vi "WSVCAP SHL Host TL RFFE Write Cycle.vi"(0 "RFFE Data Out":u8[][](array[numeric]) format="%.0x", 5 "Socket Mask":u64=1 format="%08x", 7 "Cycle CMD Lengths (bits)":u8[](array[numeric]), 9 "Cycle CMD Delay (ticks)":u32[](array[numeric]), 11 "error in":errorcluster, 13 "Log (T)":bool=TRUE, 14 "FPGA":T1) -> (15 "error out":errorcluster)   [LabVIEW 2012]
uses:
  Type Defs/WSVCAP SHL I2C FPGA Enum.ctl
  Type Defs/WSVCAP SHL Function Enum.ctl
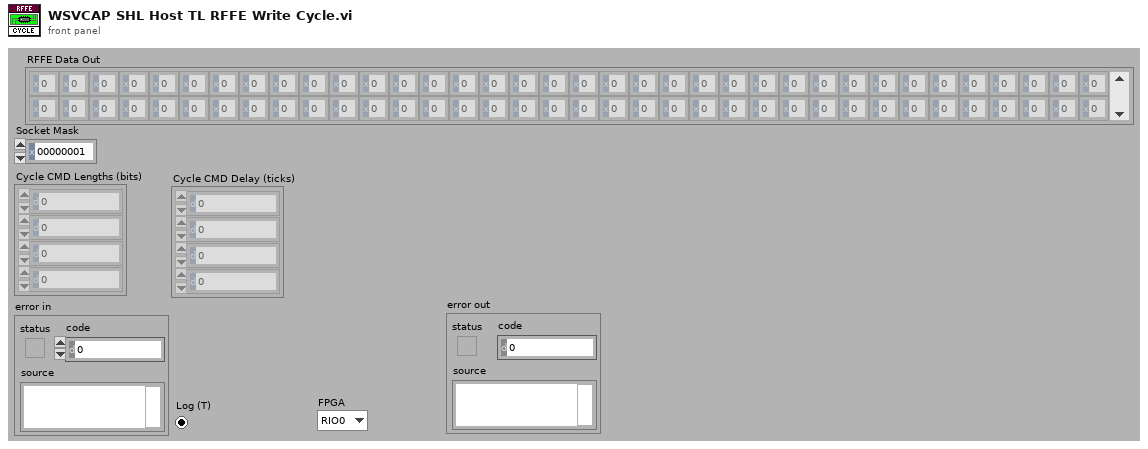
[diagram p1: front panel]
types:
  T1 = typedef "WSVCAP SHL I2C FPGA Enum.ctl" = enum16{"RIO0", "RIO1"}
  T2 = typedef "WSVCAP SHL Function Enum.ctl" = enum16{"Initialize", "Configure I2C", "Configure RFFE", "Write I2C", "Read I2C", "Write RFFE", "Read RFFE", "Start RFFE Cycle", "Stop RFFE Cycle", "Get Status", "Close"}
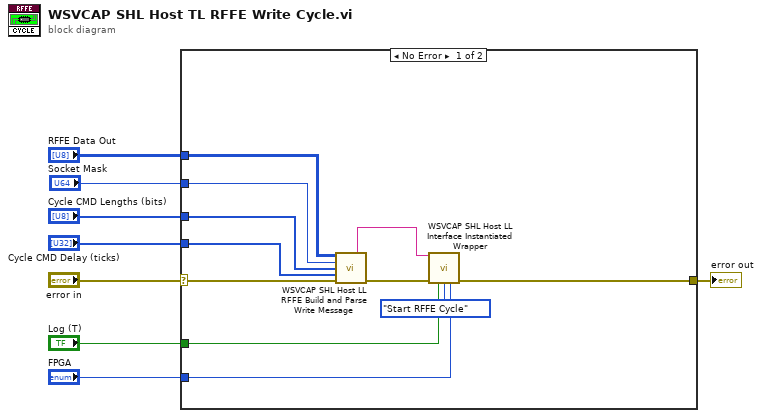
[diagram p0: block diagram]
diagram:
  n1 = case shown="No Error" "error in" {
    selector: "error in" -> [w16 w20]
    tunnel: [w10 w20] -> w8
    tunnel: "RFFE Data Out" -> [w15 _]
    tunnel: "Socket Mask" -> [w13 _]
    tunnel: "Log (T)" -> [w14 _]
    tunnel: "Cycle CMD Lengths (bits)" -> [w12 _]
    tunnel: "Cycle CMD Delay (ticks)" -> [w11 _]
    tunnel: "FPGA" -> [w9 _]
    frame No Error {
      n2 = call "WSVCAP SHL Host LL RFFE Build and Parse Write Message.vi"("Write Data In [DUT Ordered]"=w15, "Socket Mask [U64] In"=w13, "Cycle CMD Lengths (bits)"=w12, "Cycle CMD Delay (ticks)"=w11, "error in"=w16) -> ("Message Out"=w17:string, "error out"=w18:errorcluster)  [unwired: 4 in, 5 out]
      n3 = call "WSVCAP SHL Host LL Interface Instantiated Wrapper.vi"("Message In"=w17, "error in"=w18, "Log (T)"=w14, "Function"=WSVCAP_SHL_Function_Enum."Start RFFE Cycle", "FPGA"=w9) -> ("error out"=w10:errorcluster)  [unwired: 8 in, 2 out]
    }
    frame Error {
    }
  }
  "error out" <- w8
